vi "SerIO_Graph_Analog.vi"() -> ()   [LabVIEW 2013]
uses:
  <vilib>/Instr/_visa.llb/VISA Configure Serial Port (Instr).vi
panel:
  in  "Clear Chart":bool
  out "Analog Inputs":T1
  out "Analog Inputs":cluster{dbl, dbl, dbl, dbl, dbl, dbl, dbl, dbl}(graph)
  out "Current Pin & Value":i32
  out "Current Pin and Value":dbl format="%#_g mV"
  in  "Parse 2":bool
  in  "Parse":bool
  out "Serial Input Buffer":string
  in  "Stop Button":bool
  in  "VISA Name":refnum<visa-resource-name>
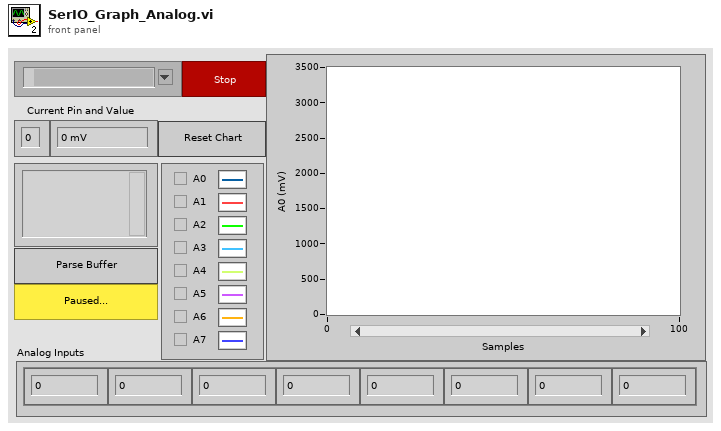
[diagram p1: front panel]
types:
  T1 = cluster{"Numeric Control":dbl, "Numeric Control":dbl, "Numeric Control":dbl, "Numeric Control":dbl, "Numeric Control":dbl, "Numeric Control":dbl, "Numeric Control":dbl, "Numeric Control":dbl}
  T2 = cluster{dbl, dbl, dbl, dbl, dbl, dbl, dbl, dbl}[]
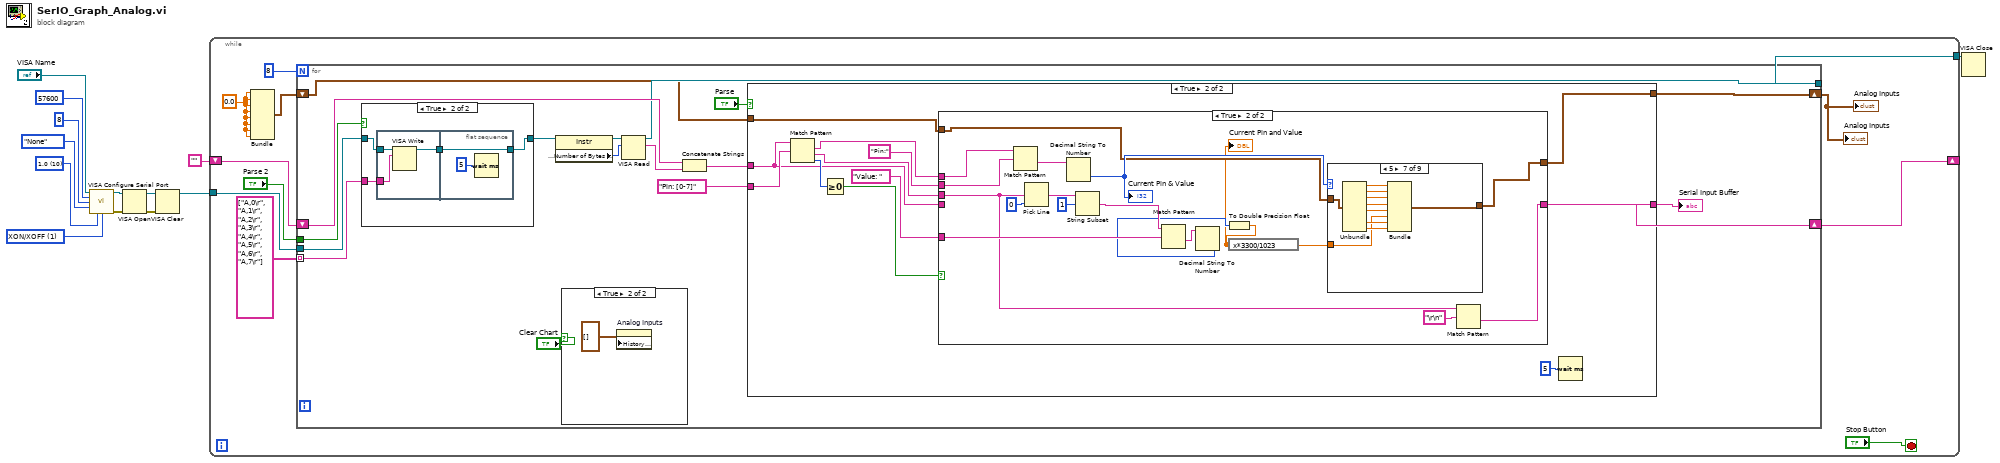
[diagram p0: block diagram]
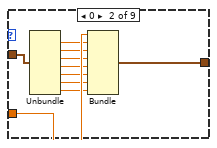
[diagram p6: hidden frame]
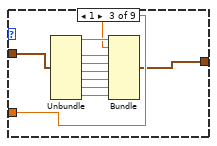
[diagram p7: hidden frame]
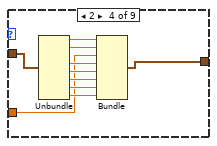
[diagram p8: hidden frame]
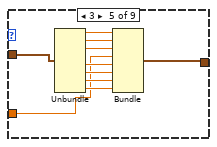
[diagram p9: hidden frame]
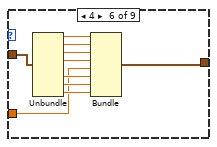
[diagram p10: hidden frame]
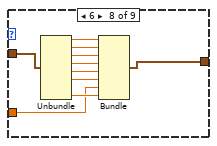
[diagram p11: hidden frame]
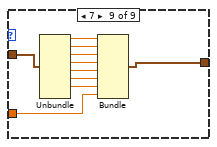
[diagram p12: hidden frame]
diagram:
  w2 = u16 1 items=["None", "XON/XOFF", "RTS/CTS", "XON/XOFF & RTS/CTS", "DTR/DSR", "XON/XOFF & DTR/DSR"] ("flow control (0:none)")
  w7 = u16 10 items=["1.0"=10, "1.5"=15, "2.0"=20] ("stop bits (10: 1 bit)")
  n1 = call-poly "VISA Configure Serial Port"("VISA resource name"="VISA Name", "baud rate (9600)"=u32 57600, "data bits (8)"=u16 8, "parity (0:none)"=enum16{"None", "Odd", "Even", "Mark", "Space"}."None", "stop bits (10: 1 bit)"=w7, "flow control (0:none)"=w2) -> ("VISA resource name out"=w11:refnum<visa-resource-name>, "error out"=w10:errorcluster)  [unwired: 8 in]
  n2 = VISA Open(error in (no error)=w10, VISA resource name=w11) -> (VISA resource name=w4:refnum<visa-resource-name>, error out=w3:errorcluster)  [unwired: 3 in]
  n3 = VISA Clear(VISA resource name=w4, error in (no error)=w3) -> (VISA resource name out=w5:refnum<visa-resource-name>)  [unwired: 1 out]
  n4 = while {
    tunnel: w5 -> [w21]
    shift-right: [w19] -> _
    shift-left: "" -> [w20]
    tunnel: [w17] -> w1
    stop <- "Stop Button" stop-if-true
    w15 = 0.0
    n5 = Bundle(w15, w15, w15, w15, w15, w15, w15, w15) -> (w16:cluster{dbl, dbl, dbl, dbl, dbl, dbl, dbl, dbl})  [unwired: 1 in]
    n6 = for {
      N: 8 -> [_]
      tunnel: string[] ["A,0\r", "A,1\r", "A,2\r", "A,3\r", "A,4\r", "A,5\r", "A,6\r", "A,7\r"] -> [w39] mode=indexing
      tunnel: w21 -> [w40]
      tunnel: "Parse 2" -> [w30]
      tunnel: [w29] -> w17
      shift-right: [w33] -> w19
      shift-left: w20 -> [w32]
      shift-right: [w26] -> w14
      shift-left: w16 -> [w27]
      n7 = case shown="True" w30 {
        tunnel: w40 -> [w157 w160]
        tunnel: w39 -> [_ w159]
        tunnel: [w157 w158] -> w38
        frame False {
        }
        frame True {
          n8 = flat-sequence {
            tunnel: w160 -> [w164]
            tunnel: w159 -> [w163]
            tunnel: [w162] -> w161
            tunnel: [w166] -> w158
            tunnel: w161 -> [w166]
            frame #0 {
              n9 = VISA Write(VISA resource name=w164, write buffer=w163) -> (VISA resource name out=w162:refnum<visa-resource-name>)  [unwired: 1 in, 2 out]
            }
            frame #1 {
              n10 = Wait (ms)(milliseconds to wait=u32 5) -> ()  [unwired: 1 out]
            }
          }
        }
      }
      n11 = property class="Instr"(reference=w38) -> (reference out=w37:refnum<visa-resource-name>, "Serial Settings:Number of Bytes at Serial Port"=w36:u32)  [unwired: 1 in, 1 out]
      n12 = case shown="True" "Clear Chart" {
        frame False {
        }
        frame True {
          n13 = property on="Analog Inputs" class="WFChart (strict)"("History Data"=T2 []) -> ()  [unwired: 2 in, 2 out]
        }
      }
      n14 = VISA Read(VISA resource name=w37, byte count=w36) -> (VISA resource name out=w29:refnum<visa-resource-name>, read buffer=w35:string)  [unwired: 1 in, 2 out]
      n15 = Concatenate Strings(w32, w35) -> (w31:string)
      n16 = case shown="True" "Parse" {
        tunnel: "Pin: [0-7]" ("regular expression") -> [_ w52]
        tunnel: [w43 w51] -> w33
        tunnel: w31 -> [w43 w50]
        tunnel: w27 -> [w42 w45]
        tunnel: [w42 w44] -> w26
        frame False {
        }
        frame True {
          n17 = Match Pattern(string=w50, regular expression=w52) -> (match substring=w53:string, after substring=w54:string, offset past match=w55:i32)  [unwired: 1 in, 1 out]
          n18 = Greater Or Equal To 0?(x=w55) -> (x >= 0?=w49:bool)
          n19 = case shown="True" w49 {
            tunnel: w54 -> [_ w65]
            tunnel: w53 -> [_ w68]
            tunnel: [w57 w64] -> w51
            tunnel: w50 -> [w57 _]
            tunnel: "Pin:" ("regular expression") -> [_ w74]
            tunnel: "Value: " ("regular expression") -> [_ w73]
            tunnel: w45 -> [w56 w62]
            tunnel: [w56 w58] -> w44
            frame False {
            }
            frame True {
              n20 = Match Pattern(string=w68, regular expression=w74) -> (after substring=w72:string)  [unwired: 1 in, 3 out]
              n21 = Pick Line(multi-line string=w65, line index=0) -> (output string=w67:string)  [unwired: 1 in]
              n22 = Decimal String To Number(string=w72) -> (number=w63:i32)  [unwired: 2 in, 1 out]
              "Current Pin & Value" <- w63
              n23 = String Subset(string=w67, offset (0)=1) -> (substring=w70:string)  [unwired: 1 in]
              n24 = Match Pattern(string=w70, regular expression=w73) -> (after substring=w71:string)  [unwired: 1 in, 3 out]
              n25 = Decimal String To Number(string=w71) -> (number=w60:i32)  [unwired: 2 in, 1 out]
              n26 = To Double Precision Float(number=w60) -> (double precision float=w59:dbl)
              "Current Pin and Value" <- w59
              n27 = expression code="x*3300/1023"(w59) -> (w61:dbl)
              n28 = case shown="5" w63 {
                tunnel: w61 -> [_ w85 w88 w98 w108 w118 w129 w139 w148]
                tunnel: w62 -> [w76 w77 w89 w99 w109 w119 w128 w138 w149]
                tunnel: [w76 w86 w87 w97 w107 w117 w127 w137 w147] -> w58
                frame -1, Default {
                }
                frame 0 {
                  n29 = Unbundle(w77) -> (w84:dbl, w83:dbl, w82:dbl, w81:dbl, w80:dbl, w79:dbl, w78:dbl)  [unwired: 1 out]
                  n30 = Bundle(w85, w84, w83, w82, w81, w80, w79, w78) -> (w86:cluster{dbl, dbl, dbl, dbl, dbl, dbl, dbl, dbl})  [unwired: 1 in]
                }
                frame 1 {
                  n31 = Unbundle(w89) -> (w90:dbl, w96:dbl, w95:dbl, w94:dbl, w93:dbl, w92:dbl, w91:dbl)  [unwired: 1 out]
                  n32 = Bundle(w90, w88, w96, w95, w94, w93, w92, w91) -> (w87:cluster{dbl, dbl, dbl, dbl, dbl, dbl, dbl, dbl})  [unwired: 1 in]
                }
                frame 2 {
                  n33 = Unbundle(w99) -> (w106:dbl, w100:dbl, w101:dbl, w102:dbl, w103:dbl, w104:dbl, w105:dbl)  [unwired: 1 out]
                  n34 = Bundle(w106, w100, w98, w101, w102, w103, w104, w105) -> (w97:cluster{dbl, dbl, dbl, dbl, dbl, dbl, dbl, dbl})  [unwired: 1 in]
                }
                frame 3 {
                  n35 = Unbundle(w109) -> (w116:dbl, w110:dbl, w111:dbl, w112:dbl, w113:dbl, w114:dbl, w115:dbl)  [unwired: 1 out]
                  n36 = Bundle(w116, w110, w111, w108, w112, w113, w114, w115) -> (w107:cluster{dbl, dbl, dbl, dbl, dbl, dbl, dbl, dbl})  [unwired: 1 in]
                }
                frame 4 {
                  n37 = Unbundle(w119) -> (w126:dbl, w120:dbl, w121:dbl, w122:dbl, w123:dbl, w124:dbl, w125:dbl)  [unwired: 1 out]
                  n38 = Bundle(w126, w120, w121, w122, w118, w123, w124, w125) -> (w117:cluster{dbl, dbl, dbl, dbl, dbl, dbl, dbl, dbl})  [unwired: 1 in]
                }
                frame 5 {
                  n39 = Unbundle(w128) -> (w136:dbl, w130:dbl, w131:dbl, w132:dbl, w133:dbl, w134:dbl, w135:dbl)  [unwired: 1 out]
                  n40 = Bundle(w136, w130, w131, w132, w133, w129, w134, w135) -> (w127:cluster{dbl, dbl, dbl, dbl, dbl, dbl, dbl, dbl})  [unwired: 1 in]
                }
                frame 6 {
                  n41 = Unbundle(w138) -> (w140:dbl, w146:dbl, w145:dbl, w144:dbl, w143:dbl, w142:dbl, w141:dbl)  [unwired: 1 out]
                  n42 = Bundle(w140, w146, w145, w144, w143, w142, w139, w141) -> (w137:cluster{dbl, dbl, dbl, dbl, dbl, dbl, dbl, dbl})  [unwired: 1 in]
                }
                frame 7 {
                  n43 = Unbundle(w149) -> (w150:dbl, w156:dbl, w155:dbl, w154:dbl, w153:dbl, w152:dbl, w151:dbl)  [unwired: 1 out]
                  n44 = Bundle(w150, w156, w155, w154, w153, w152, w151, w148) -> (w147:cluster{dbl, dbl, dbl, dbl, dbl, dbl, dbl, dbl})  [unwired: 1 in]
                }
              }
              n45 = Match Pattern(string=w65, regular expression="\r\n") -> (after substring=w64:string)  [unwired: 1 in, 3 out]
            }
          }
          n46 = Wait (ms)(milliseconds to wait=u32 5) -> ()  [unwired: 1 out]
        }
      }
      "Serial Input Buffer" <- w33
    }
    "Analog Inputs" <- w14
    "Analog Inputs" <- w14
  }
  n47 = VISA Close(VISA resource name=w1) -> ()  [unwired: 1 in, 1 out]
